vi "Error_Control_Brass.vi"(0 "ERD Loop":refnum<queue>, 1 "GEA2":refnum<queue>, 2 "Command (Handle Errors)":T1=enum."Handle Errors", 5 "Receive Loop":refnum<user-event>, 7 "UI Loop Error":refnum<user-event>, 11 "Error In":errorcluster, 12 "Cont Send":refnum<queue>) -> (15 "Error Out":errorcluster)   [LabVIEW 2016]
uses:
  type defs2/Error_Command_Brass.ctl
  type defs2/ERD_Data_Loop_Control_Brass.ctl
  type defs2/ERD_Loop_States_Brass.ctl
  Common/GExplorer Support/typedefs/GExplorer_Data_Cluster.ctl
  type defs2/Cont_Send_States_Brass.ctl
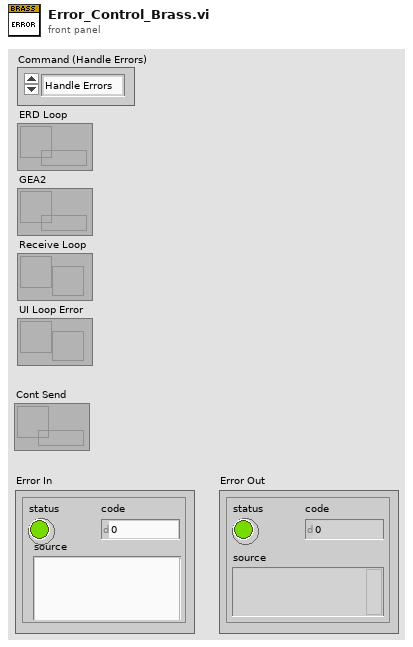
[diagram p1: front panel]
types:
  T1 = typedef "Error_Command_Brass.ctl" = enum16{"Initialize", "Handle Errors", "Report Errors"}
  T2 = typedef "Cont_Send_States_Brass.ctl" = enum16{"Run", "Shutdown"}
  T3 = typedef "ERD_Data_Loop_Control_Brass.ctl" = cluster{"Data":variant, "State":T4}
  T4 = typedef "ERD_Loop_States_Brass.ctl" = enum16{"Init", "Build ERD Read List", "Read ERDs", "Update UI", "Update Graphs", "Read Faults", "Log Data", "Pause", "Shutdown"}
  T5 = typedef "GExplorer_Data_Cluster.ctl" = cluster{"Data":variant, "State":enum16{"Add to Log", "Clear", "Shutdown"}}
  T6 = typedef "Ref_ReceiveLoop_UserEvent.ctl" = refnum<user-event>
  T7 = typedef "Ref_UILoop_UserEvent.ctl" = refnum<user-event>
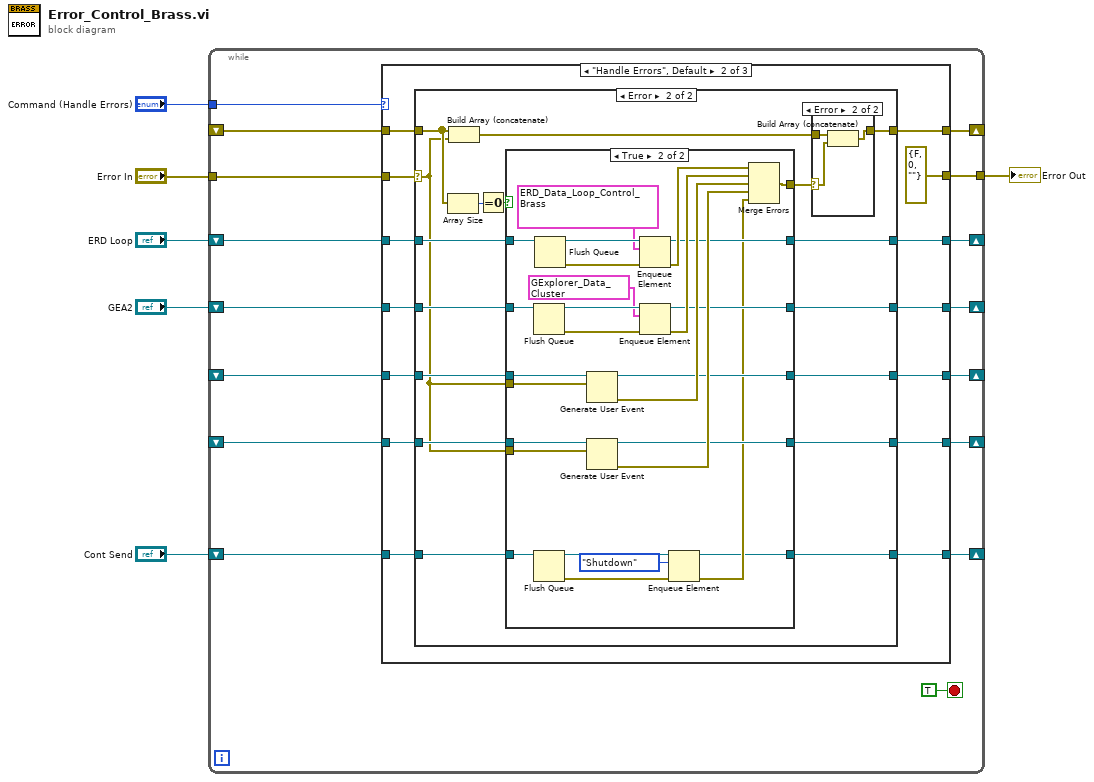
[diagram p0: block diagram]
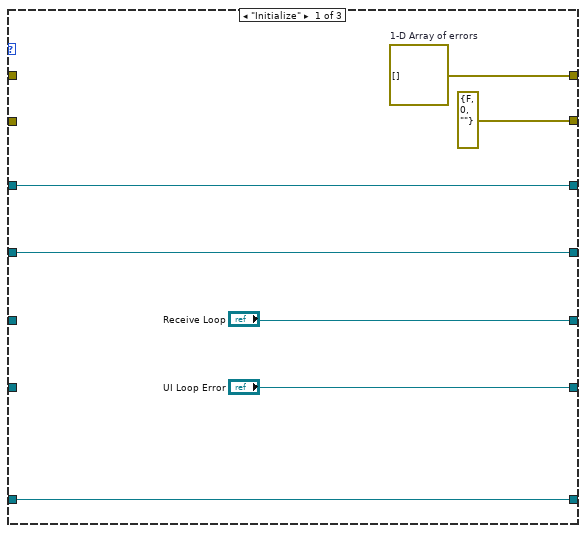
[diagram p2: hidden frame]
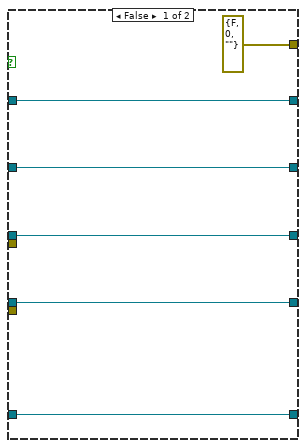
[diagram p4: hidden frame]
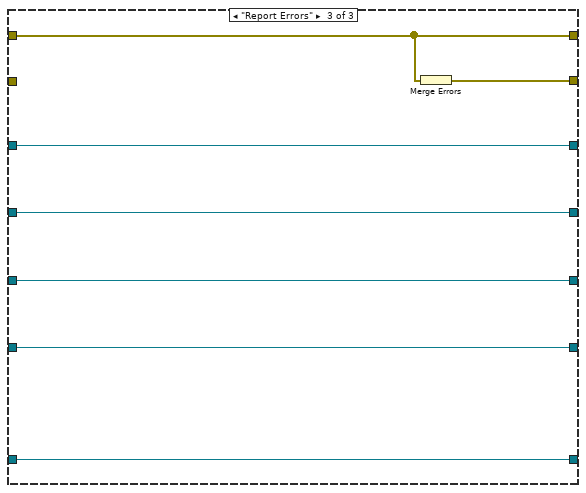
[diagram p6: hidden frame]
diagram:
  n1 = while {
    tunnel: "Error In" -> [w20]
    tunnel: "Command (Handle Errors)" -> [w21]
    shift-right: [w19] -> _
    shift-left: _ -> [w18]
    tunnel: [w17] -> w4
    shift-right: [w16] -> _
    shift-left: "ERD Loop" -> [w12]
    shift-right: [w15] -> _
    shift-left: "GEA2" -> [w11]
    shift-right: [w14] -> _
    shift-left: _ -> [w10]
    shift-right: [w13] -> _
    shift-left: _ -> [w9]
    shift-right: [w8] -> _
    shift-left: "Cont Send" -> [w7]
    stop <- TRUE stop-if-true
    n2 = case shown="\"Handle Errors\", Default" w21 {
      tunnel: w20 -> [_ w43 _]
      tunnel: [w29 w37 w109] -> w19
      tunnel: w18 -> [_ w42 w109]
      tunnel: [errorcluster {"status"=FALSE, "code"=0, "source"=""} ("Error In") errorcluster {"status"=FALSE, "code"=0, "source"=""} ("Error In") w110] -> w17
      tunnel: [w27 w35 w108] -> w16
      tunnel: [w26 w36 w107] -> w15
      tunnel: ["Receive Loop" w34 w106] -> w14
      tunnel: ["UI Loop Error" w33 w105] -> w13
      tunnel: w12 -> [w27 w41 w108]
      tunnel: w11 -> [w26 w40 w107]
      tunnel: w10 -> [_ w39 w106]
      tunnel: w9 -> [_ w38 w105]
      tunnel: [w23 w30 w104] -> w8
      tunnel: w7 -> [w23 w31 w104]
      frame "Initialize" {
        w29 = errorcluster[] []  # 1-D Array of errors
      }
      frame "Handle Errors", Default {
        n3 = case shown="Error" w43 {
          selector: w43 -> [_ w57]
          tunnel: w42 -> [w49 w66]
          tunnel: w41 -> [w48 w63]
          tunnel: w40 -> [w47 w62]
          tunnel: w39 -> [w46 w61]
          tunnel: w38 -> [w45 w60]
          tunnel: [w49 w58] -> w37
          tunnel: [w47 w56] -> w36
          tunnel: [w48 w55] -> w35
          tunnel: [w46 w54] -> w34
          tunnel: [w45 w53] -> w33
          tunnel: w31 -> [w44 w51]
          tunnel: [w44 w50] -> w30
          frame No Error {
          }
          frame Error {
            n4 = Array Size(array=w66) -> (size(s)=w65:i32)
            n5 = Build Array (concatenate)(w66, w57) -> (w52:errorcluster[])
            n6 = Equal To 0?(x=w65) -> (x = 0?=w64:bool)
            n7 = case shown="True" w64 {
              tunnel: w63 -> [w71 w99]
              tunnel: w62 -> [w70 w98]
              tunnel: w61 -> [w69 w90]
              tunnel: w60 -> [w68 w88]
              tunnel: [errorcluster {"status"=FALSE, "code"=0, "source"=""} ("error IO") w97] -> w59
              tunnel: w57 -> [_ w89]
              tunnel: w57 -> [_ w87]
              tunnel: [w70 w82] -> w56
              tunnel: [w71 w81] -> w55
              tunnel: [w69 w80] -> w54
              tunnel: [w68 w79] -> w53
              tunnel: w51 -> [w67 w78]
              tunnel: [w67 w73] -> w50
              frame False {
              }
              frame True {
                n8 = Flush Queue(queue=w98) -> (queue out=w95:refnum<queue>, error out=w96:errorcluster)  [unwired: 1 in, 1 out]
                n9 = Flush Queue(queue=w78) -> (queue out=w76:refnum<queue>, error out=w77:errorcluster)  [unwired: 1 in, 1 out]
                n10 = Flush Queue(queue=w99) -> (queue out=w92:refnum<queue>, error out=w93:errorcluster)  [unwired: 1 in, 1 out]
                n11 = Generate User Event(user event=w90, event data cluster=w89) -> (user event out=w80:T6, error out=w85:errorcluster)  [unwired: 2 in]
                n12 = Generate User Event(user event=w88, event data cluster=w87) -> (user event out=w79:T7, error out=w86:errorcluster)  [unwired: 2 in]
                n13 = Enqueue Element(queue=w92, element=T3 {"Data"=variant, "State"=enum."Shutdown"}, error in (no error)=w93) -> (queue out=w81:refnum<queue>, error out=w84:errorcluster)  [unwired: 1 in, 1 out]
                n14 = Enqueue Element(queue=w95, element=T5 {"Data"=variant, "State"=enum."Shutdown"}, error in (no error)=w96) -> (queue out=w82:refnum<queue>, error out=w83:errorcluster)  [unwired: 1 in, 1 out]
                n15 = Enqueue Element(queue=w76, element=Cont_Send_States_Brass."Shutdown", error in (no error)=w77) -> (queue out=w73:refnum<queue>, error out=w74:errorcluster)  [unwired: 1 in, 1 out]
                n16 = Merge Errors(w84, w83, w85, w86, w74) -> (w97:errorcluster)
              }
            }
            n17 = case shown="Error" w59 {
              selector: w59 -> [_ w102]
              tunnel: [w100 w103] -> w58
              tunnel: w52 -> [w100 w101]
              frame No Error {
              }
              frame Error {
                n18 = Build Array (concatenate)(w101, w102) -> (w103:errorcluster[])
              }
            }
          }
        }
      }
      frame "Report Errors" {
        n19 = Merge Errors(w109) -> (w110:errorcluster)
      }
    }
  }
  "Error Out" <- w4
